vi "test Create Messages Nonintegral State.vi"(8 "error in (no error)":errorcluster, 11 "TestCase in":refnum<class "Routing and Faulting Unit Tests.lvclass">) -> (0 "error out":errorcluster, 3 "TestCase out":refnum<class "Routing and Faulting Unit Tests.lvclass">)   [LabVIEW 2017, in "Routing and Faulting Unit Tests.lvclass"]
uses:
  Routing and Faulting Unit Tests.lvclass
  Engine/Engine Data.ctl
  Shared/Compiled.Settings.ctl
  Shared/Communication Configuration.ctl
  Shared/Routing and Faulting Configuration.ctl
  Shared/Routing Channel Configuration.ctl
  Shared/Value-Connections Map.ctl
  Shared/Alias Mapping.ctl
  Shared/Compiled Connection.ctl
  Shared/FIFO Indices.ctl
  Includes/CDMessaging.lvlibp/Producer/Abstract Producer/Abstract Producer.lvclass
  Engine/Device Inputs.ctl
  Engine/Device Outputs.ctl
  <vilib>/addons/_JKI Toolkits/VI Tester/TestCase.llb/TestCase.lvclass
  Engine/Routing and Faulting Engine.lvlib
  Shared/Routing and Faulting Shared.lvlib
  C:/Program Files (x86)/National Instruments/LabVIEW 2017/vi.lib/addons/_JKI Toolkits/VI Tester/TestCase.llb/TestCase.lvclass
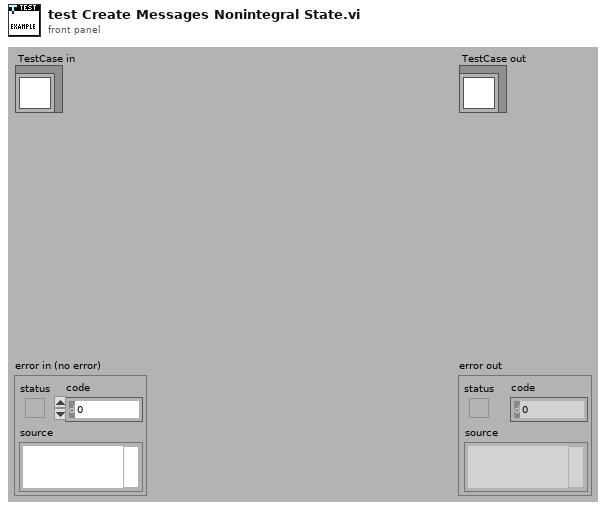
[diagram p1: front panel]
types:
  T1 = typedef "Routing and Faulting Shared.lvlib/Routing Channel Configuration.ctl" = cluster{"Channel Name":string, "Initial Value":dbl, "FIFO Index":i32, "Value-Connections Map":T2}
  T2 = typedef "Routing and Faulting Shared.lvlib/Value-Connections Map.ctl" = cluster{"State Value Array":i32[], "Connection List Array":cluster{"Compiled Connections Indices":i32[]}[]}
  T3 = typedef "Routing and Faulting Shared.lvlib/Compiled Connection.ctl" = cluster{"Consumer Queue Index":i32, "Normalized Connection String":string}
  T4 = typedef "Routing and Faulting Shared.lvlib/Communication Configuration.ctl" = cluster{"Consumer Queue Names":string[], "Resource Names":string[]}
  T5 = typedef "Routing and Faulting Shared.lvlib/Routing and Faulting Configuration.ctl" = cluster{"Routing Channel Configurations":T1[], "Alias Mappings":T6[], "Compiled Connection Buffer":T3[]}
  T6 = typedef "Routing and Faulting Shared.lvlib/Alias Mapping.ctl" = cluster{"Endpoint":string, "Alias":string}
  T7 = typedef "Routing and Faulting Engine.lvlib/Engine Data.ctl" = cluster{"Compiled.Settings":T8, "Producer":refnum<class "Abstract Producer.lvclass">, "Device Inputs":T10, "Device Outputs":T11, "States Changed":bool[]}
  T8 = typedef "Routing and Faulting Shared.lvlib/Compiled.Settings.ctl" = cluster{"Custom Device Name":string, "Communication Configuration":T4, "Routing and Faulting Configuration":T5, "Status Channels FIFO Indices":T9}
  T9 = typedef "Routing and Faulting Shared.lvlib/FIFO Indices.ctl" = cluster{"Status Channel":i32, "Heartbeat Channel":i32}
  T10 = typedef "Routing and Faulting Engine.lvlib/Device Inputs.ctl" = cluster{"Current Inputs":dbl[], "Previous Inputs":dbl[], "Device Inputs FIFO":refnum<k33>}
  T11 = typedef "Routing and Faulting Engine.lvlib/Device Outputs.ctl" = cluster{"Outputs":dbl[], "Device Outputs FIFO":refnum<k33>}
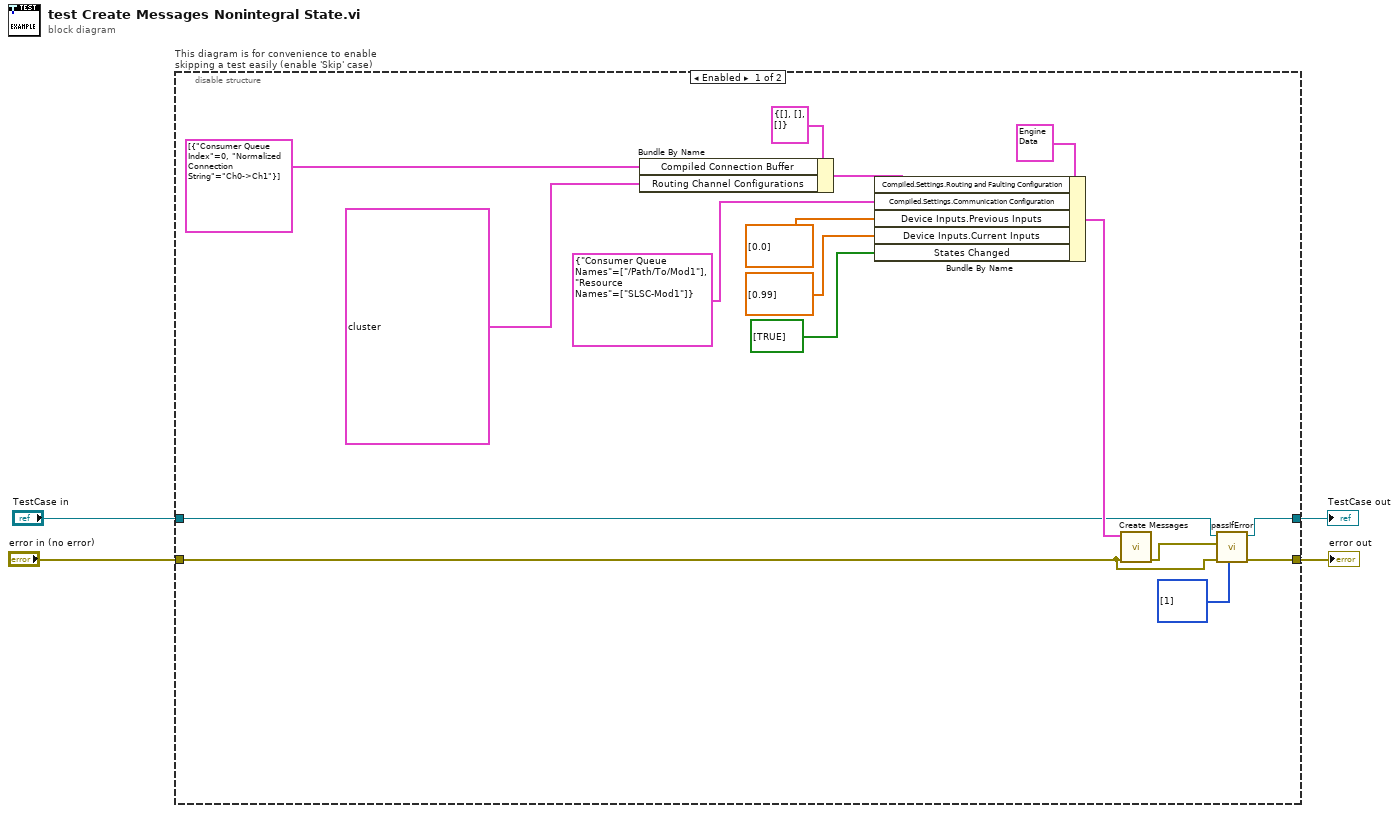
[diagram p0: block diagram]
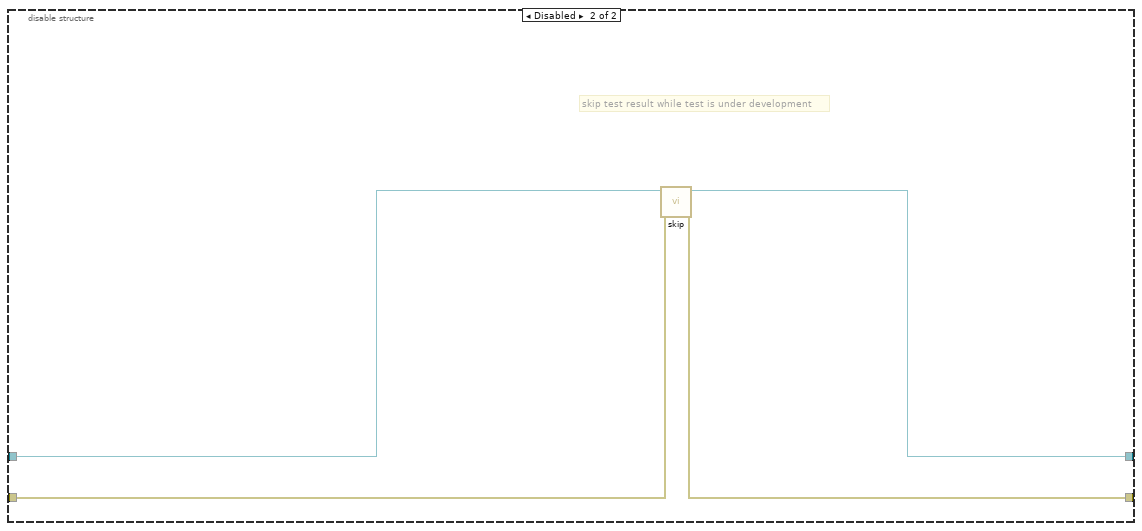
[diagram p2: hidden frame]
diagram:
  n1 = disable-structure "This diagram is for convenience to enable skipping a test easily (enable 'Skip' case)" shown="Enabled" {
    disable-tunnel: "TestCase in" -> [w7 w24]
    disable-tunnel: [w6 w22] -> w1
    disable-tunnel: [w10 w23] -> w3
    disable-tunnel: "error in (no error)" -> [w9 w21]
    frame Enabled {
      n2 = Bundle By Name(cluster=T5 {"Routing Channel Configurations"=[], "Alias Mappings"=[], "Compiled Connection Buffer"=[]} ("Compiled.Settings.Routing and Faulting Configuration"), "Compiled Connection Buffer"=T3[] [{"Consumer Queue Index"=0, "Normalized Connection String"="Ch0->Ch1"}], "Routing Channel Configurations"=T1[] [{"Channel Name"="Window Up", "Initial Value"=0.0, "FIFO Index"=0, "Value-Connections Map"={"State Value Array"=[0, 1], "Connection List Array"=[{"Compiled Connections Indices"=[]}, {"Compiled Connections Indices"=[0]}]}}]) -> (w18:T5)
      n3 = Bundle By Name(cluster=T7 {"Compiled.Settings"={"Custom Device Name"="", "Communication Configuration"={"Consumer Queue Names"=[], "Resource Names"=[]}, "Routing and Faulting Configuration"={"Routing Channel Configurations"=[], "Alias Mappings"=[], "Compiled Connection Buffer"=[]}, "Status Channels FIFO Indices"={"Status Channel"=0, "Heartbeat Channel"=0}}, "Producer"=refnum, "Device Inputs"={"Current Inputs"=[], "Previous Inputs"=[], "Device Inputs FIFO"=refnum}, "Device Outputs"={"Outputs"=[], "Device Outputs FIFO"=refnum}, "States Changed"=[]} ("Engine Data in"), "Compiled.Settings.Routing and Faulting Configuration"=w18, "Compiled.Settings.Communication Configuration"=T4 {"Consumer Queue Names"=["/Path/To/Mod1"], "Resource Names"=["SLSC-Mod1"]}, "Device Inputs.Previous Inputs"=dbl[] [0.0] ("State Value Array"), "Device Inputs.Current Inputs"=dbl[] [0.99] ("State Value Array"), "States Changed"=bool[] [TRUE]) -> (w14:T7)
      n4 = call "Create Messages.vi"("error in (no error)"=w9, "Engine Data in"=w14) -> ("error out"=w8:errorcluster)  [unwired: 6 in, 3 out]
      n5 = call-dynamic "passIfError.vi"("passing error codes (default = any error code)"=i32[] [1], "error in (no error)"=w9, "error"=w8, "TestCase in"=w7) -> ("error out"=w10:errorcluster, "TestCase out"=w6:refnum<class "Routing and Faulting Unit Tests.lvclass">)  [unwired: 6 in]
    }
    frame Disabled {
      # "skip test result while test is under development"
      n6 = call <vilib>:"skip.vi"("error in (no error)"=w21, "TestCase in"=w24) -> ("error out"=w23:errorcluster, "TestCase out"=w22:refnum<class "Routing and Faulting Unit Tests.lvclass">)  [unwired: 8 in]
    }
  }
  "error out" <- w3
  "TestCase out" <- w1
